vi "selectAutonMode.vi"(2 "Auton File":dbl) -> ()   [LabVIEW 2011]
uses:
  Robot Global Data.vi
panel:
  out "Auton Array":dbl[][](array[numeric])
  out "Current File":string
  in  "Auton Files":string[](array[string])
  in  "Number of Auton Files":dbl
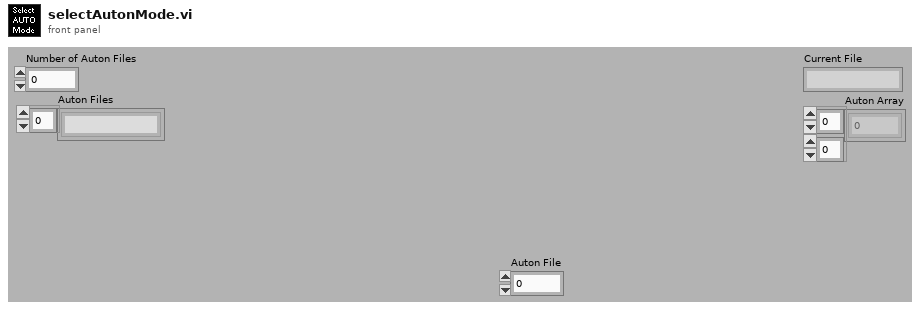
[diagram p1: front panel]
types:
  T1 = enum16{"False", "FalseToTrue", "True", "TrueToFalse"}
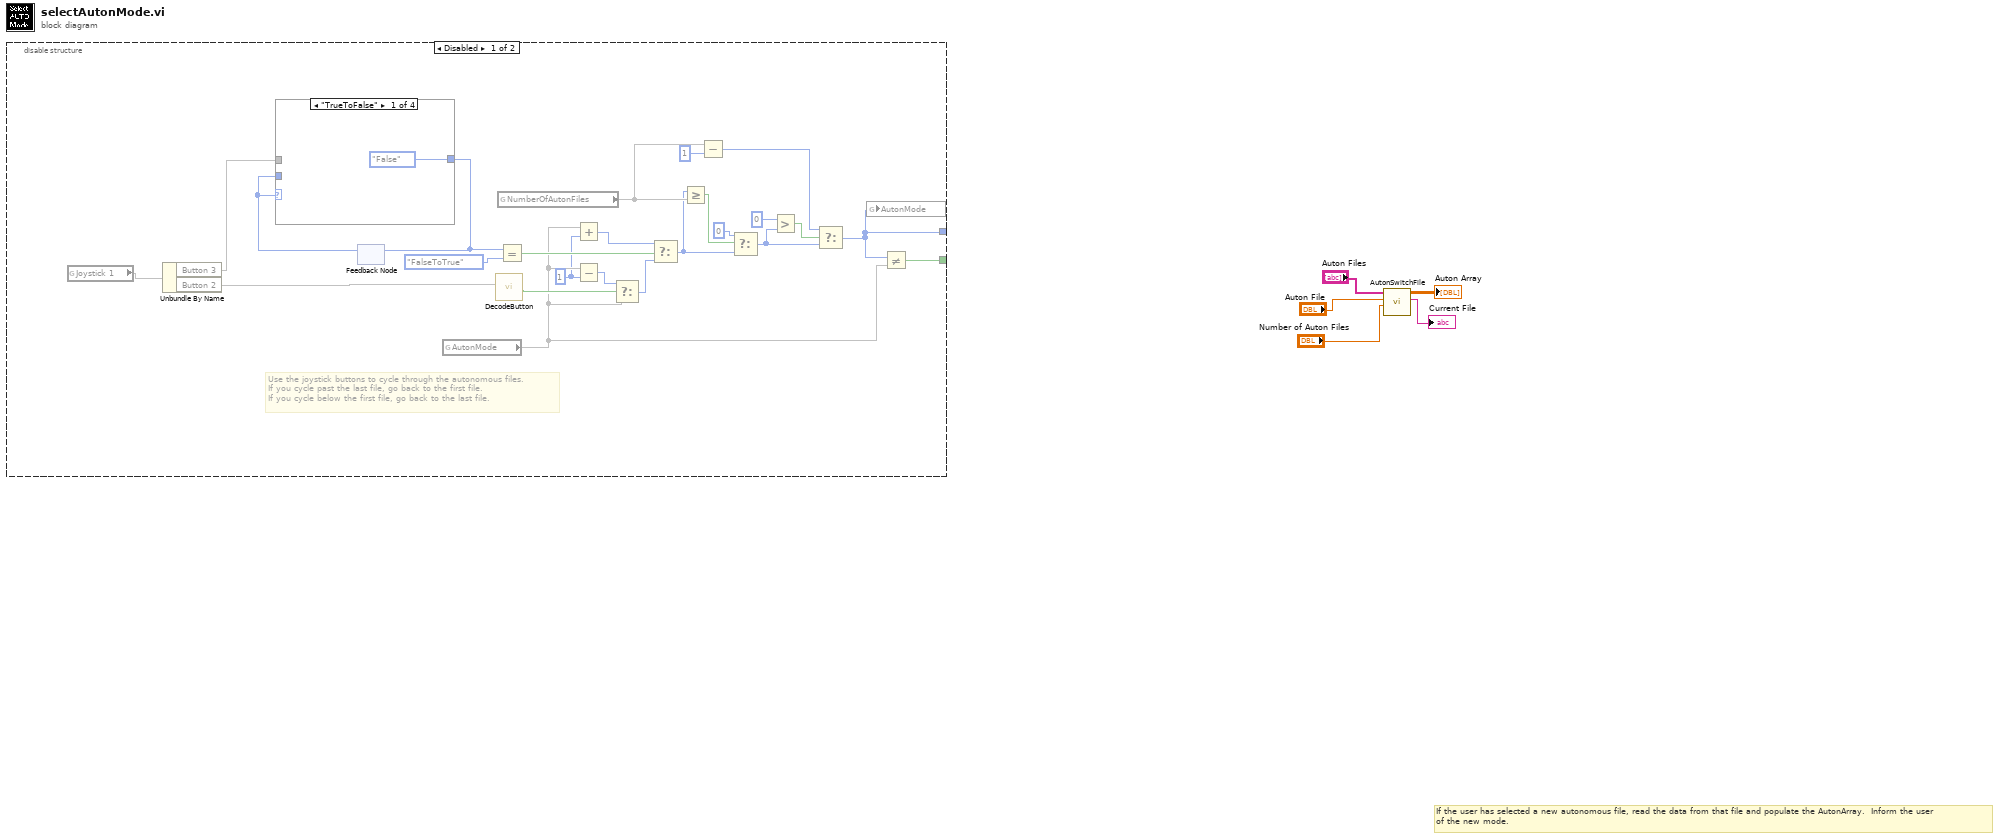
[diagram p0: block diagram]
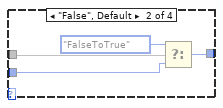
[diagram p2: hidden frame]
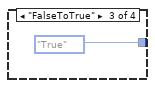
[diagram p3: hidden frame]
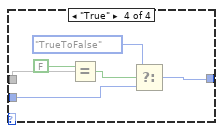
[diagram p4: hidden frame]
diagram:
  # "If the user has selected a new autonomous file, read the data from that file and populate the AutonArray.  Inform the user\nof the new mode."
  n1 = disable-structure shown="Disabled" {
    disable-tunnel: [w29 _] -> _
    disable-tunnel: [w19 _] -> _
    frame Disabled {
      w10 = i16 1 ("y")
      # "Use the joystick buttons to cycle through the autonomous files.\nIf you cycle past the last file, go back to the first file.\nIf you cycle below the first file, go back to the last file."
      n2 = global read "Robot Global Data.vi" "Joystick 1"() -> (w6)
      n3 = Unbundle By Name(w6) -> ("Button 3"=w17, "Button 2"=w7)
      n4 = feedback #1() -> (w14:T1)  [unwired: 1 out]
      n5 = case shown="\"TrueToFalse\"" w14 {
        tunnel: w17 -> [_ w34 _ w40]
        tunnel: [T1."False" ("f") w32 T1."True" ("y") w41] -> w15
        tunnel: w14 -> [_ w31 _ w37]
        frame "TrueToFalse" {
        }
        frame "False", Default {
          n6 = Select(t=T1."FalseToTrue", s=w34, f=w31) -> (s? t:f=w32:T1)
        }
        frame "FalseToTrue" {
        }
        frame "True" {
          n7 = Equal?(x=FALSE, y=w40) -> (x = y?=w38:bool)
          n8 = Select(t=T1."TrueToFalse", s=w38, f=w37) -> (s? t:f=w41:T1)
        }
      }
      n9 = feedback-in #1(w15) -> ()
      n10 = global read "Robot Global Data.vi" "AutonMode"() -> (w12)
      n11 = call "DecodeButton.vi"("Button"=w7) -> ("False to True"=w13:bool)  [unwired: 10 out]
      n12 = global read "Robot Global Data.vi" "NumberOfAutonFiles"() -> (w26)
      n13 = Equal?(x=w15, y=T1."FalseToTrue") -> (x = y?=w18:bool)
      n14 = Add(x=w12, y=w10) -> (x+y=w11:i16)
      n15 = Subtract(x=w12, y=w10) -> (x-y=w8:i16)
      n16 = Select(t=w8, s=w13, f=w12) -> (s? t:f=w9:i16)
      n17 = Select(t=w11, s=w18, f=w9) -> (s? t:f=w20:i16)
      n18 = Greater Or Equal?(x=w20, y=w26) -> (x >= y?=w21:bool)
      n19 = Subtract(x=w26, y=i16 1) -> (x-y=w28:i16)
      n20 = Select(t=i16 0, s=w21, f=w20) -> (s? t:f=w23:i16)
      n21 = Greater?(x=i16 0, y=w23) -> (0:w25:bool)
      n22 = Select(t=w28, s=w25, f=w23) -> (s? t:f=w29:i16)
      n23 = global write "Robot Global Data.vi" "AutonMode"(w29) -> ()
      n24 = Not Equal?(x=w29, y=w12) -> (x != y?=w19:bool)
    }
    frame Enabled {
    }
  }
  n25 = call "AutonSwitchFile.vi"("Number of Auton Files"="Number of Auton Files", "Auton File"="Auton File", "Auton Files"="Auton Files") -> ("Current File"=→"Current File":string, "Auton Array"=→"Auton Array":dbl[][])  [unwired: 7 in]
